vi "dingshipanduan.vi"(0 "i":i32, 1 "心率":dbl) -> (2 "测试结果":string, 3 "正常":bool, 4 "报警":bool, 5 "开始":bool)   [LabVIEW 2016]
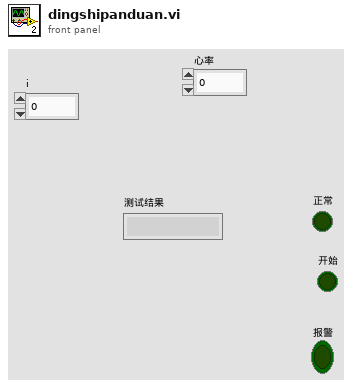
[diagram p1: front panel]
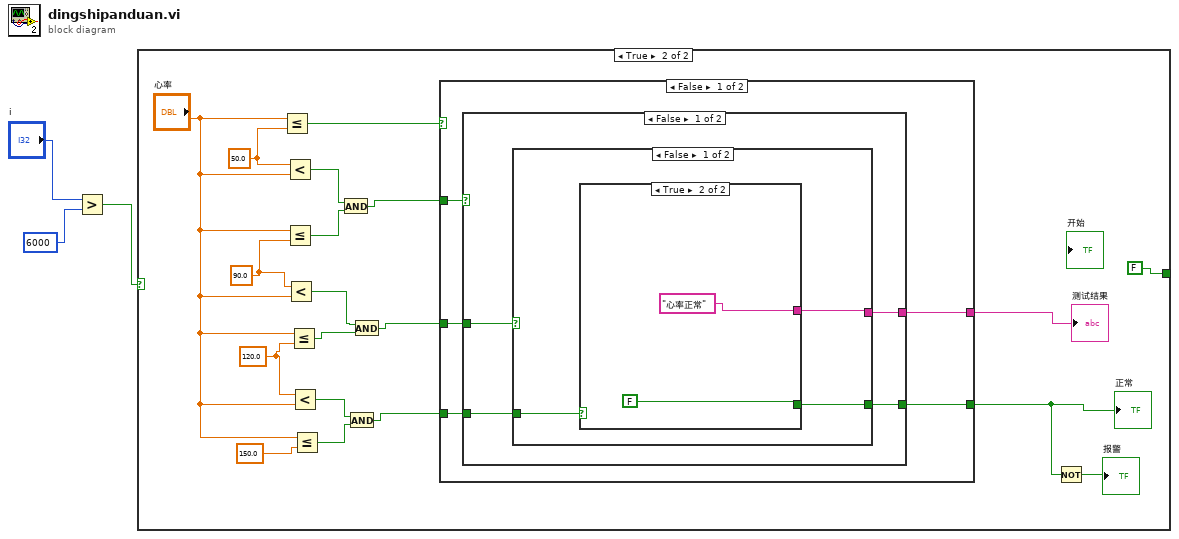
[diagram p0: block diagram]
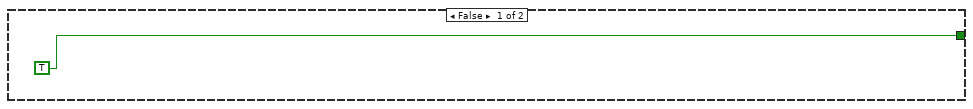
[diagram p2: hidden frame]
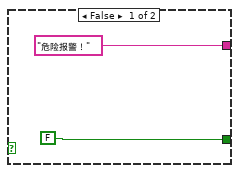
[diagram p3: hidden frame]
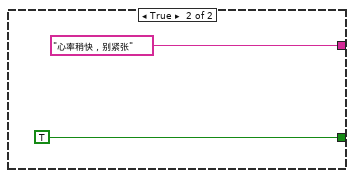
[diagram p4: hidden frame]
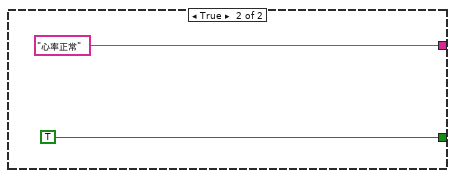
[diagram p5: hidden frame]
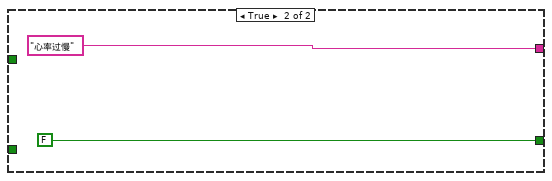
[diagram p6: hidden frame]
diagram:
  n1 = Greater?(x="i", y=6000) -> (0:w1:bool)
  n2 = case shown="True" w1 {
    tunnel: [TRUE FALSE] -> _
    frame False {
    }
    frame True {
      w21 = 120.0
      w20 = 90.0
      w23 = 50.0
      n3 = Less Or Equal?(x="心率", y=w23) -> (x <= y?=w18:bool)
      n4 = Less?(x=w23, y="心率") -> (x < y?=w17:bool)
      n5 = Less Or Equal?(x="心率", y=w20) -> (x <= y?=w16:bool)
      n6 = Less?(x=w20, y="心率") -> (x < y?=w14:bool)
      n7 = Less Or Equal?(x="心率", y=w21) -> (x <= y?=w13:bool)
      n8 = Less?(x=w21, y="心率") -> (x < y?=w11:bool)
      n9 = Less Or Equal?(x="心率", y=150.0) -> (x <= y?=w10:bool)
      n10 = And(x=w17, y=w16) -> (x .and. y?=w15:bool)
      n11 = And(x=w11, y=w10) -> (x .and. y?=w9:bool)
      n12 = And(x=w14, y=w13) -> (x .and. y?=w12:bool)
      n13 = case shown="False" w18 {
        tunnel: w15 -> [w28 _]
        tunnel: w12 -> [w27 _]
        tunnel: w9 -> [w26 _]
        tunnel: [w25 FALSE] -> w6
        tunnel: [w24 "心率过慢"] -> w5
        frame False {
          n14 = case shown="False" w28 {
            tunnel: w27 -> [w32 _]
            tunnel: w26 -> [w31 _]
            tunnel: [w30 TRUE] -> w25
            tunnel: [w29 "心率正常"] -> w24
            frame False {
              n15 = case shown="False" w32 {
                tunnel: w31 -> [w35 _]
                tunnel: [w34 TRUE] -> w30
                tunnel: [w33 "心率稍快，别紧张"] -> w29
                frame False {
                  n16 = case shown="True" w35 {
                    tunnel: [FALSE FALSE] -> w34
                    tunnel: ["危险报警！" "心率正常"] -> w33
                    frame False {
                    }
                    frame True {
                    }
                  }
                }
                frame True {
                }
              }
            }
            frame True {
            }
          }
        }
        frame True {
        }
      }
      "正常" <- w6
      "测试结果" <- w5
      n17 = Not(x=w6) -> (.not. x?=→"报警":bool)
    }
  }
